vi "Fetch IQ Recorder Measurement IQ Amplitudes.vi"(8 "error in (no error)":errorcluster, 10 "Instance (1)":i32=1 format="%.0g", 11 "VISA resource name":refnum<visa-resource-name>) -> (0 "error out":errorcluster, 1 "Q Amplitudes":dbl[](array[numeric]) format="%.2p", 2 "I Amplitudes":dbl[](array[numeric]) format="%.2p", 3 "VISA resource name out":refnum<visa-resource-name>, 5 "Reliability":i32)   [LabVIEW 2020, in "Rohde&Schwarz CMXP GPRF.lvlib"]
doc: "Returns the I and Q amplitudes.\n\nAttribute:\nRSCMXPGPRF_ATTR_FETCH_IQ_RECORDER_MEASUREMENT_IQ_AMPLITUDES\n\nRemote-control command:\nFETCh:GPRF:MEAS<i>:IQRecorder?"
uses:
  <instrlib>/Rohde&Schwarz CMXP GPRF/Rohde&Schwarz CMXP GPRF.lvlib
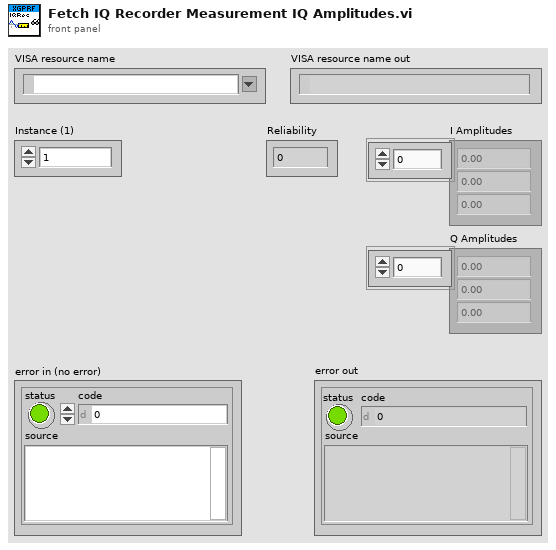
[diagram p1: front panel]
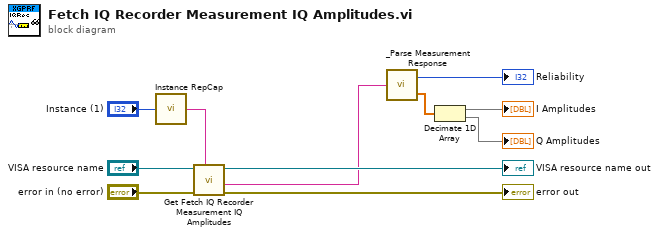
[diagram p0: block diagram]
diagram:
  n1 = call <instrlib>:"Instance RepCap.vi"("Instance in"="Instance (1)") -> ("Instance out"=w11:string)
  n2 = call "Get Fetch IQ Recorder Measurement IQ Amplitudes"("Repeated Capabilities"=w11, "error in (no error)"="error in (no error)", "instrument handle"="VISA resource name") -> ("error out"=→"error out":errorcluster, "Fetch IQ Recorder Measurement IQ Amplitudes"=w1:string, "instrument handle out"=→"VISA resource name out":refnum<visa-resource-name>)  [unwired: 6 in]
  n3 = call <instrlib>:"_Parse Measurement Response.vi"("String In"=w1) -> ("Reliability"=→"Reliability":i32, "Data"=w2:dbl[])
  n4 = Decimate 1D Array(w2) -> (→"I Amplitudes":dbl[], →"Q Amplitudes":dbl[])
